vi "g_ECS02_Command.vi"() -> ()   [LabVIEW 2014]
panel:
  in  "Response":string
  in  "Send":bool
  in  "Command":string
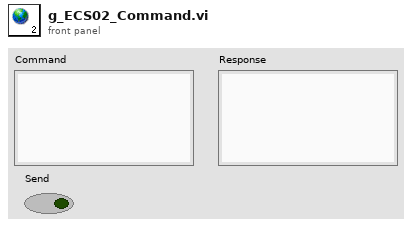
[diagram p1: front panel]
diagram:
